vi "Lab Panel V5.25.vi"() -> ()   [LabVIEW 2017] (continued)
                n199 = local write "LAB03 TEMP"(w225) -> ()
                n200 = Unbundle(w202) -> ("id1"=→"LAB01-TP":bool, "id2"=→"LAB02-TP":bool, "id3"=→"LAB03-TP":bool, "id4"=→"LAB04-TP":bool, "id5"=→"LAB05-TP":bool)
                n201 = local read "TEMP LA05"() -> (w210:T9)
                n202 = local read "TEMP LA04"() -> (w217:T9)
                n203 = local read "TEMP LA02"() -> (w231:T9)
                n204 = local read "TEMP LA03"() -> (w224:T9)
                n205 = local read "TEMP LA01"() -> (w238:T9)
                n206 = Bundle(cluster=w224, "TL-1"=w222, "TN-1"=w221, "TL-2"=w220, "TN-2"=w219) -> (w223:T9)  [unwired: 4 in]
                n207 = Bundle(cluster=w238, "TL-1"=w237, "TN-1"=w236, "TL-2"=w235, "TN-2"=w234) -> (w233:T9)  [unwired: 4 in]
                n208 = Bundle(cluster=w231, "TL-1"=w229, "TN-1"=w228, "TL-2"=w227, "TN-2"=w226) -> (w230:T9)  [unwired: 4 in]
                n209 = Bundle(cluster=w217, "TL-1"=w216, "TN-1"=w215, "TL-2"=w214, "TN-2"=w213) -> (w212:T9)  [unwired: 4 in]
                n210 = Bundle(cluster=w210, "TL-1"=w209, "TN-1"=w208, "TL-2"=w207, "TN-2"=w206) -> (w205:T9)  [unwired: 4 in]
                n211 = local write "TEMP LA03"(w223) -> ()
                n212 = local write "TEMP LA01"(w233) -> ()
                n213 = local write "TEMP LA02"(w230) -> ()
                n214 = local write "TEMP LA05"(w205) -> ()
                n215 = local write "TEMP LA04"(w212) -> ()
              }
            }
            frame #2 {
              w252 = 0
              n216 = local read "LAB01 TEMP"() -> (w254:T12)
              n217 = local read "SIG LAB01-2"() -> (w249:T2)
              n218 = Unbundle By Name(w254) -> ("T1 Live"=w247:dbl, "T1 Neut"=w246:dbl, "T2 Live"=w245:dbl, "T2 Neut"=w244:dbl)  [unwired: 2 out]
              n219 = local read "SIG LAB01-1"() -> (w251:T2)
              n220 = local read "TEMP LA01"() -> (w255:T9)
              n221 = Bundle By Name(cluster=w255, "TL-1"=w247, "TN-1"=w246, "TL-2"=w245, "TN-2"=w244, "TL -1COUNT"=w252, "TN-1 COUNT"=w252, "TL-2 COUNT"=w252, "TN-2 COUNT"=w252) -> (w253:T9)
              n222 = Bundle(cluster=w251, "Tmp Live"=w247, "Tmp Neut"=w246) -> (w250:T2)  [unwired: 3 in]
              n223 = Bundle(cluster=w249, "Tmp Live"=w245, "Tmp Neut"=w244) -> (w248:T2)  [unwired: 3 in]
              n224 = local write "SIG LAB01-2"(w248) -> ()
              n225 = local write "SIG LAB01-1"(w250) -> ()
              n226 = local write "TEMP LA01"(w253) -> ()
            }
            frame #3 {
              w264 = 0
              n227 = local read "LAB02 TEMP"() -> (w266:T12)
              n228 = Unbundle By Name(w266) -> ("T1 Live"=w259:dbl, "T1 Neut"=w258:dbl, "T2 Live"=w257:dbl, "T2 Neut"=w256:dbl)  [unwired: 2 out]
              n229 = local read "SIG LAB02-1"() -> (w263:T2)
              n230 = local read "SIG LAB02-2"() -> (w262:T2)
              n231 = local read "TEMP LA02"() -> (w267:T9)
              n232 = Bundle By Name(cluster=w267, "TL-1"=w259, "TN-1"=w258, "TL-2"=w257, "TN-2"=w256, "TL -1COUNT"=w264, "TN-1 COUNT"=w264, "TL-2 COUNT"=w264, "TN-2 COUNT"=w264) -> (w265:T9)
              n233 = Bundle(cluster=w262, "Tmp Live"=w257, "Tmp Neut"=w256) -> (w260:T2)  [unwired: 3 in]
              n234 = Bundle(cluster=w263, "Tmp Live"=w259, "Tmp Neut"=w258) -> (w261:T2)  [unwired: 3 in]
              n235 = local write "TEMP LA02"(w265) -> ()
              n236 = local write "SIG LAB02-1"(w261) -> ()
              n237 = local write "SIG LAB02-2"(w260) -> ()
            }
            frame #4 {
              w276 = 0
              n238 = local read "LAB03 TEMP"() -> (w278:T12)
              n239 = Unbundle By Name(w278) -> ("T1 Live"=w271:dbl, "T1 Neut"=w270:dbl, "T2 Live"=w269:dbl, "T2 Neut"=w268:dbl)  [unwired: 2 out]
              n240 = local read "SIG LAB03-1"() -> (w275:T2)
              n241 = local read "SIG LAB03-2"() -> (w274:T2)
              n242 = local read "TEMP LA03"() -> (w279:T9)
              n243 = Bundle By Name(cluster=w279, "TL-1"=w271, "TN-1"=w270, "TL-2"=w269, "TN-2"=w268, "TL -1COUNT"=w276, "TN-1 COUNT"=w276, "TL-2 COUNT"=w276, "TN-2 COUNT"=w276) -> (w277:T9)
              n244 = Bundle(cluster=w274, "Tmp Live"=w269, "Tmp Neut"=w268) -> (w272:T2)  [unwired: 3 in]
              n245 = Bundle(cluster=w275, "Tmp Live"=w271, "Tmp Neut"=w270) -> (w273:T2)  [unwired: 3 in]
              n246 = local write "TEMP LA03"(w277) -> ()
              n247 = local write "SIG LAB03-2"(w272) -> ()
              n248 = local write "SIG LAB03-1"(w273) -> ()
            }
            frame #5 {
              w288 = 0
              n249 = local read "LAB04 TEMP"() -> (w290:T12)
              n250 = Unbundle By Name(w290) -> ("T1 Live"=w283:dbl, "T1 Neut"=w282:dbl, "T2 Live"=w281:dbl, "T2 Neut"=w280:dbl)  [unwired: 2 out]
              n251 = local read "SIG LAB04-2"() -> (w286:T2)
              n252 = local read "SIG LAB04-1"() -> (w287:T2)
              n253 = local read "TEMP LA04"() -> (w291:T9)
              n254 = Bundle By Name(cluster=w291, "TL-1"=w283, "TN-1"=w282, "TL-2"=w281, "TN-2"=w280, "TL -1COUNT"=w288, "TN-1 COUNT"=w288, "TL-2 COUNT"=w288, "TN-2 COUNT"=w288) -> (w289:T9)
              n255 = Bundle(cluster=w286, "Tmp Live"=w281, "Tmp Neut"=w280) -> (w284:T2)  [unwired: 3 in]
              n256 = Bundle(cluster=w287, "Tmp Live"=w283, "Tmp Neut"=w282) -> (w285:T2)  [unwired: 3 in]
              n257 = local write "SIG LAB04-2"(w284) -> ()
              n258 = local write "TEMP LA04"(w289) -> ()
              n259 = local write "SIG LAB04-1"(w285) -> ()
            }
            frame #6 {
              w300 = 0
              n260 = local read "LAB05 TEMP"() -> (w302:T12)
              n261 = Unbundle By Name(w302) -> ("T1 Live"=w295:dbl, "T1 Neut"=w294:dbl, "T2 Live"=w293:dbl, "T2 Neut"=w292:dbl)  [unwired: 2 out]
              n262 = local read "SIG LAB05-2"() -> (w298:T2)
              n263 = local read "SIG LAB05-1"() -> (w299:T2)
              n264 = local read "TEMP LA05"() -> (w303:T9)
              n265 = Bundle By Name(cluster=w303, "TL-1"=w295, "TN-1"=w294, "TL-2"=w293, "TN-2"=w292, "TL -1COUNT"=w300, "TN-1 COUNT"=w300, "TL-2 COUNT"=w300, "TN-2 COUNT"=w300) -> (w301:T9)
              n266 = Bundle(cluster=w298, "Tmp Live"=w293, "Tmp Neut"=w292) -> (w296:T2)  [unwired: 3 in]
              n267 = Bundle(cluster=w299, "Tmp Live"=w295, "Tmp Neut"=w294) -> (w297:T2)  [unwired: 3 in]
              n268 = local write "SIG LAB05-2"(w296) -> ()
              n269 = local write "SIG LAB05-1"(w297) -> ()
              n270 = local write "TEMP LA05"(w301) -> ()
            }
          }
        }
        frame #10 {
          # "create analog task"
          n271 = local read "AI Task0"() -> (w310:dbl)
          n272 = local read "AI Task1"() -> (w309:dbl)
          n273 = local read "AI Task2"() -> (w308:dbl)
          n274 = call "sub vi - AI USB4704 (3)  Create Task v2.vi"("Task In 0"=w310, "Task In 1"=w309, "Task In 2"=w308) -> ("TASK USB 0"=→"AI Task0":i32, "TASK USB 1"=→"AI Task1":i32, "TASK USB 2"=→"AI Task2":i32, "AI Task Er"=→"AI Task":bool)  [unwired: 8 in, 1 out]
        }
        frame #11 {
          # "enable front panel, all settings done"
          n275 = property on="Tab Control 2" class="TabCtl (strict)"("DisabledEnum"=T16."Enabled" ("Disabled")) -> ()  [unwired: 2 in, 2 out]
          n276 = property on="Tab Control 2" class="TabCtl (strict)"("Value"=0) -> ()  [unwired: 2 in, 2 out]
        }
        frame #12 {
          n277 = property on="Tab Control 2" class="TabCtl (strict)"("Value"=0) -> ()  [unwired: 2 in, 2 out]
        }
      }
    }
    frame #2 {
      n278 = node-c288("loop  delay(mS)") -> (w316:T18)  [unwired: 3 in]
      n279 = timed-loop {
        timing: w316 -> [_]
        timing-out: [_] -> w315
        i -> [w342]
        stop <- w317 stop-if-true
        n280 = node-c288() -> ()  [unwired: 1 in, 1 out]
        n281 = local read "Resets Done"() -> (w321:dbl)
        n282 = Greater?(x=w321, y=50) -> (0:w318:bool)
        n283 = local read "SELECT LAB05-2"() -> (w322:T3)
        n284 = local read "SELECT LAB05-1"() -> (w323:T3)
        n285 = local read "SELECT LAB04-2"() -> (w324:T3)
        n286 = Or(x=w318, y="stop") -> (x .or. y?=w317:bool)
        n287 = local read "SELECT LAB03-1"() -> (w327:T3)
        n288 = local read "SELECT LAB02-2"() -> (w328:T3)
        n289 = local read "SELECT LAB01-1"() -> (w331:T3)
        n290 = local read "SELECT LAB03-2"() -> (w326:T3)
        n291 = local read "SELECT LAB01-2"() -> (w330:T3)
        n292 = local read "SELECT LAB04-1"() -> (w325:T3)
        n293 = local read "SELECT LAB02-1"() -> (w329:T3)
        n294 = local read "run lab03-2"() -> (w336:bool)
        n295 = local read "run lab04-1"() -> (w335:bool)
        n296 = local read "run lab05-1"() -> (w333:bool)
        n297 = local read "run lab04-2"() -> (w334:bool)
        n298 = local read "run lab05-2"() -> (w332:bool)
        n299 = local read "run lab03-1"() -> (w337:bool)
        n300 = local read "run lab02-2"() -> (w338:bool)
        n301 = local read "run lab02-1"() -> (w339:bool)
        n302 = local read "run lab01-1"() -> (w341:bool)
        n303 = local read "run lab01-2"() -> (w340:bool)
        n304 = global write "Global display 1.vi" "stop disp"(w317) -> ()
        n305 = stacked-sequence {
          seq-local: [_ w408 _ _ _ _ _ _ _ _ _ _ _ _ _ _ _ _ _ _ _ _ _ _] -> [_ _ _ _ _ w2509 _ _ _ _ _ _ _ _ _ _ _ _ _ _ _ _ _ _]
          seq-local: [_ w407 _ _ _ _ _ _ _ _ _ _ _ _ _ _ _ _ _ _ _ _ _ _] -> [_ _ _ _ _ w2508 _ _ _ _ _ _ _ _ _ _ _ _ _ _ _ _ _ _]
          seq-local: [_ w394 _ _ _ _ _ _ _ _ _ _ _ _ _ _ _ _ _ _ _ _ _ _] -> [_ _ _ _ _ w2507 _ _ _ _ _ _ _ _ _ _ _ _ _ _ _ _ _ _]
          seq-local: [_ w393 _ _ _ _ _ _ _ _ _ _ _ _ _ _ _ _ _ _ _ _ _ _] -> [_ _ _ _ _ w2506 _ _ _ _ _ _ _ _ _ _ _ _ _ _ _ _ _ _]
          seq-local: [_ w392 _ _ _ _ _ _ _ _ _ _ _ _ _ _ _ _ _ _ _ _ _ _] -> [_ _ _ _ _ w2505 _ _ _ _ _ _ _ _ _ _ _ _ _ _ _ _ _ _]
          seq-local: [_ w391 _ _ _ _ _ _ _ _ _ _ _ _ _ _ _ _ _ _ _ _ _ _] -> [_ _ _ _ _ w2504 _ _ _ _ _ _ _ _ _ _ _ _ _ _ _ _ _ _]
          seq-local: [_ w390 _ _ _ _ _ _ _ _ _ _ _ _ _ _ _ _ _ _ _ _ _ _] -> [_ _ _ _ _ w2503 _ _ _ _ _ _ _ _ _ _ _ _ _ _ _ _ _ _]
          seq-local: [_ w389 _ _ _ _ _ _ _ _ _ _ _ _ _ _ _ _ _ _ _ _ _ _] -> [_ _ _ _ _ w2502 _ _ _ _ _ _ _ _ _ _ _ _ _ _ _ _ _ _]
          seq-local: [_ w388 _ _ _ _ _ _ _ _ _ _ _ _ _ _ _ _ _ _ _ _ _ _] -> [_ _ _ _ _ w2501 _ _ _ _ _ _ _ _ _ _ _ _ _ _ _ _ _ _]
          seq-local: [_ w387 _ _ _ _ _ _ _ _ _ _ _ _ _ _ _ _ _ _ _ _ _ _] -> [_ _ _ _ _ w2500 _ _ _ _ _ _ _ _ _ _ _ _ _ _ _ _ _ _]
          seq-local: [_ _ _ _ _ _ _ _ _ _ _ w3640 _ _ _ _ _ _ _ _ _ _ _ _] -> [_ _ _ _ _ _ _ _ _ _ _ _ w3661 _ _ _ _ _ _ _ _ _ _ _]
          tunnel: w341 -> [_ _ w424 w672 w2099 w2529 w2844 w3331 _ _ _ _ _ w3946 _ w4903 _ _ w5190 w5493 w5674 _ _ _]
          tunnel: w340 -> [_ _ w423 w670 w2098 w2528 w2845 w3330 _ _ _ _ _ w3945 _ w4901 _ _ w5189 w5492 w5672 _ _ _]
          tunnel: w339 -> [_ _ w422 w668 w2097 w2527 w2843 w3329 _ _ _ _ _ w3944 _ w4899 _ _ w5188 w5491 w5671 _ _ _]
          tunnel: w338 -> [_ _ w421 w666 w2096 w2526 w2842 w3328 _ _ _ _ _ w3943 _ w4897 _ _ w5187 w5490 w5670 _ _ _]
          tunnel: w337 -> [_ _ w420 w664 w2095 w2525 w2841 w3327 _ _ _ _ _ w3942 _ w4895 _ _ w5186 w5489 w5669 _ _ _]
          tunnel: w336 -> [_ _ w419 w662 w2094 w2524 w2840 w3326 _ _ _ _ _ w3941 _ w4893 _ _ w5185 w5488 w5668 _ _ _]
          tunnel: w335 -> [_ _ w418 w660 w2093 w2523 w2839 w3325 _ _ _ _ _ w3940 _ w4891 _ _ w5184 w5487 w5667 _ _ _]
          tunnel: w334 -> [_ _ w417 w658 w2092 w2522 w2838 w3324 _ _ _ _ _ w3939 _ w4889 _ _ w5183 w5486 w5666 _ _ _]
          tunnel: w333 -> [_ _ w416 w656 w2091 w2521 w2837 w3323 _ _ _ _ _ w3938 _ w4887 _ _ w5182 w5485 w5665 _ _ _]
          tunnel: w332 -> [_ _ w415 w654 w2090 w2520 w2836 w3322 _ _ _ _ _ w3937 _ w4885 _ _ w5181 w5484 w5664 _ _ _]
          tunnel: w331 -> [_ _ _ w671 w2089 w2519 _ _ _ _ _ _ _ _ _ w4905 _ _ _ _ _ w6018 _ _]
          tunnel: w330 -> [_ _ _ w669 w2088 w2518 _ _ _ _ _ _ _ _ _ w4900 _ _ _ _ _ w6017 _ _]
          tunnel: w329 -> [_ _ _ w667 w2087 w2517 _ _ _ _ _ _ _ _ _ w4898 _ _ _ _ _ w6016 _ _]
          tunnel: w328 -> [_ _ _ w665 w2086 w2516 _ _ _ _ _ _ _ _ _ w4896 _ _ _ _ _ w6015 _ _]
          tunnel: w327 -> [_ _ _ w663 w2085 w2515 _ _ _ _ _ _ _ _ _ w4894 _ _ _ _ _ w6014 _ _]
          tunnel: w326 -> [_ _ _ w661 w2084 w2514 _ _ _ _ _ _ _ _ _ w4892 _ _ _ _ _ w6013 _ _]
          tunnel: w325 -> [_ _ _ w659 w2083 w2513 _ _ _ _ _ _ _ _ _ w4890 _ _ _ _ _ w6012 _ _]
          tunnel: w324 -> [_ _ _ w657 w2082 w2512 _ _ _ _ _ _ _ _ _ w4888 _ _ _ _ _ w6011 _ _]
          tunnel: w323 -> [_ _ _ w655 w2081 w2511 _ _ _ _ _ _ _ _ _ w4886 _ _ _ _ _ w6010 _ _]
          tunnel: w322 -> [_ _ _ w653 w2080 w2510 _ _ _ _ _ _ _ _ _ w4884 _ _ _ _ _ w6009 _ _]
          tunnel: w318 -> [_ _ _ _ _ _ _ _ _ _ _ _ _ _ _ _ _ _ _ _ _ _ _ w6071]
          tunnel: w317 -> [_ _ _ _ _ _ _ _ _ _ _ _ _ _ _ _ _ _ _ _ _ _ _ w6070]
          frame #0 {
            w350 = FALSE
            w355 = 0.5
            # "set up cycle control"
            n306 = local read "jig cycle"() -> (w354:dbl)
            n307 = local read "Amps Fail level"() -> (w348:dbl)
            n308 = local read "Simulate"() -> (w345:bool)
            n309 = Divide(x="JIG ON TIME (S)", y=w355) -> (x/y=→"on loops":dbl)
            n310 = Divide(x="JIG OFF TIME (S)", y=w355) -> (x/y=→"off loops":dbl)
            n311 = Increment(x=w354) -> (x+1=w353:dbl)
            n312 = local write "Simulate IND"(w345) -> ()
            n313 = global write "Global display 3.vi" "Amps Fail"(w348) -> ()
            n314 = local write "TEMP"(w350) -> ()
            n315 = local write "AI"(w350) -> ()
            n316 = local read "Network Directory"() -> (w347:path)
            n317 = local write "jig cycle"(w353) -> ()
            n318 = call "sub vi - check network dir v2.vi"("PATH"=w347) -> ("error"=w346:bool)  [unwired: 10 in]
            n319 = local write "network error"(w346) -> ()
            n320 = global write "Global display 3.vi" "network drive"(w346) -> ()
            n321 = event shown="[1] \"ADMIN\": Value Change" {
              selector: _ -> [_ _]
              dyn-events: _ -> [_ _]
              timeout: 10 -> [_ _]
              event Timeout {
                n322 = event-data() -> ()  [unwired: 1 in, 3 out]
              }
              event "ADMIN": Value Change {
                n323 = event-data() -> ()  [unwired: 1 in, 6 out]
                n324 = stacked-sequence {
                  seq-local: [_ w359 _] -> [_ _ w360]
                  frame #0 {
                    n325 = global write "Global 1.vi" "password"("9949") -> ()
                  }
                  frame #1 {
                    n326 = call "sub vi - password 1.vi"() -> ("RESULT"=w359:bool)  [unwired: 11 in]
                  }
                  frame #2 {
                    w362 = FALSE
                    n327 = property on="Tab Control 2" class="TabCtl (strict)"() -> ("Pages"=w366:refnum<vi>[])  [unwired: 2 in, 2 out]
                    n328 = Select(t=TRUE, s=w360, f=w362) -> (s? t:f=w361:bool)
                    n329 = Index Array(array=w366, index=8) -> (element=w364:refnum<vi>)
                    n330 = property class="Page"(reference=w364, "PageVis"=w361) -> ()  [unwired: 1 in, 2 out]
                    n331 = local write "ADMIN"(w362) -> ()
                  }
                }
              }
            }
          }
          frame #1 {
            w404 = 60.0
            # "convert temperature rise minutes to cycles"
            n332 = local read "SET LAB05-2"() -> (w368:T5)
            n333 = local read "SET LAB05-1"() -> (w370:T5)
            n334 = local read "SET LAB04-2"() -> (w372:T5)
            n335 = local read "SET LAB01-1"() -> (w386:T5)
            n336 = local read "SET LAB01-2"() -> (w384:T5)
            n337 = local read "SET LAB02-2"() -> (w380:T5)
            n338 = local read "SET LAB04-1"() -> (w374:T5)
            n339 = local read "SET LAB03-1"() -> (w378:T5)
            n340 = local read "SET LAB03-2"() -> (w376:T5)
            n341 = local read "SET LAB02-1"() -> (w382:T5)
            n342 = local read "JIG OFF TIME (S)"() -> (w409:dbl)
            n343 = local read "JIG ON TIME (S)"() -> (w410:dbl)
            n344 = Unbundle(w368) -> ("T-RISE mins"=w367:dbl)  [unwired: 4 out]
            n345 = Unbundle(w370) -> ("T-RISE mins"=w369:dbl)  [unwired: 4 out]
            n346 = Unbundle(w386) -> ("T-RISE mins"=w385:dbl)  [unwired: 4 out]
            n347 = Unbundle(w372) -> ("T-RISE mins"=w371:dbl)  [unwired: 4 out]
            n348 = Unbundle(w384) -> ("T-RISE mins"=w383:dbl)  [unwired: 4 out]
            n349 = Unbundle(w382) -> ("T-RISE mins"=w381:dbl)  [unwired: 4 out]
            n350 = Unbundle(w374) -> ("T-RISE mins"=w373:dbl)  [unwired: 4 out]
            n351 = Unbundle(w380) -> ("T-RISE mins"=w379:dbl)  [unwired: 4 out]
            n352 = Unbundle(w376) -> ("T-RISE mins"=w375:dbl)  [unwired: 4 out]
            n353 = Unbundle(w378) -> ("T-RISE mins"=w377:dbl)  [unwired: 4 out]
            n354 = Add(x=w410, y=w409) -> (x+y=w403:dbl)
            n355 = Multiply(x=w404, y=w375) -> (x*y=w399:dbl)
            n356 = Multiply(x=w404, y=w373) -> (x*y=w398:dbl)
            n357 = Multiply(x=w404, y=w371) -> (x*y=w397:dbl)
            n358 = Multiply(x=w404, y=w369) -> (x*y=w396:dbl)
            n359 = Multiply(x=w404, y=w367) -> (x*y=w395:dbl)
            n360 = Multiply(x=w404, y=w383) -> (x*y=w405:dbl)
            n361 = Multiply(x=w404, y=w377) -> (x*y=w400:dbl)
            n362 = Multiply(x=w404, y=w385) -> (x*y=w406:dbl)
            n363 = Multiply(x=w404, y=w381) -> (x*y=w402:dbl)
            n364 = Multiply(x=w404, y=w379) -> (x*y=w401:dbl)
            n365 = Divide(x=w396, y=w403) -> (x/y=w388:dbl)
            n366 = Divide(x=w397, y=w403) -> (x/y=w389:dbl)
            n367 = Divide(x=w398, y=w403) -> (x/y=w390:dbl)
            n368 = Divide(x=w395, y=w403) -> (x/y=w387:dbl)
            n369 = Divide(x=w400, y=w403) -> (x/y=w392:dbl)
            n370 = Divide(x=w406, y=w403) -> (x/y=w408:dbl)
            n371 = Divide(x=w405, y=w403) -> (x/y=w407:dbl)
            n372 = Divide(x=w402, y=w403) -> (x/y=w394:dbl)
            n373 = Divide(x=w401, y=w403) -> (x/y=w393:dbl)
            n374 = Divide(x=w399, y=w403) -> (x/y=w391:dbl)
          }
          frame #2 {
            # "control cycle loops"
            n375 = local read "JIG OFF TIME (S)"() -> (w413:dbl)
            n376 = local read "JIG ON TIME (S)"() -> (w412:dbl)
            n377 = local read "jig cycle"() -> (w426:dbl)
            n378 = local read "on loops"() -> (w428:dbl)
            n379 = local read "off loops"() -> (w427:dbl)
            n380 = Add(x=w413, y=w412) -> (x+y=w411:dbl)
            n381 = Add(x=w428, y=w427) -> (x+y=w414:dbl)
            n382 = Greater Or Equal?(x=w426, y=w414) -> (x >= y?=w425:bool)
            n383 = case shown="True" w425 {
              tunnel: w424 -> [_ w462]
              tunnel: w423 -> [_ w461]
              tunnel: w422 -> [_ w460]
              tunnel: w421 -> [_ w459]
              tunnel: w420 -> [_ w458]
              tunnel: w419 -> [_ w457]
              tunnel: w418 -> [_ w456]
              tunnel: w417 -> [_ w455]
              tunnel: w416 -> [_ w454]
              tunnel: w415 -> [_ w453]
              tunnel: w411 -> [_ w452]
              frame False {
              }
              frame True {
                # "increment cycle value and convert cycles to minutes for temp rise"
                n384 = stacked-sequence {
                  frame #0 {
                    n385 = local read "Temp read loop"() -> (w465:dbl)
                    n386 = Increment(x=w465) -> (x+1=w464:dbl)
                    n387 = local write "Temp read loop"(w464) -> ()
                  }
                  frame #1 {
                    n388 = local read "Temp read loop"() -> (w466:dbl)
                    n389 = Greater?(x=w466, y=20) -> (0:w468:bool)
                    n390 = case shown="True" w468 {
                      frame False {
                      }
                      frame True {
                        n391 = local write "Temp read loop"(1) -> ()
                      }
                    }
                  }
                }
                n392 = local read "JIG RELAY CYCLES"() -> (w451:T8)
                n393 = local read "Temp read loop"() -> (→"Tp Up":dbl)
                n394 = Unbundle By Name(w451) -> ("LAB01-1"=w449:dbl, "LAB01-2"=w447:dbl, "LAB02-1"=w445:dbl, "LAB02-2"=w443:dbl, "LAB03-1"=w441:dbl, "LAB03-2"=w439:dbl, "LAB04-1"=w437:dbl, "LAB04-2"=w435:dbl, "LAB05-1"=w433:dbl, "LAB05-2"=w431:dbl)
                n395 = stacked-sequence {
                  tunnel: w462 -> [w480 _ _ _ _ _ _ _ _ _]
                  tunnel: w461 -> [_ w497 _ _ _ _ _ _ _ _]
                  tunnel: w460 -> [_ _ w514 _ _ _ _ _ _ _]
                  tunnel: w459 -> [_ _ _ w531 _ _ _ _ _ _]
                  tunnel: w458 -> [_ _ _ _ w548 _ _ _ _ _]
                  tunnel: w457 -> [_ _ _ _ _ w565 _ _ _ _]
                  tunnel: w456 -> [_ _ _ _ _ _ w582 _ _ _]
                  tunnel: w455 -> [_ _ _ _ _ _ _ w599 _ _]
                  tunnel: w454 -> [_ _ _ _ _ _ _ _ w616 _]
                  tunnel: w453 -> [_ _ _ _ _ _ _ _ _ w633]
                  tunnel: w452 -> [w477 w494 w511 w528 w545 w562 w579 w596 w613 w630]
                  tunnel: w449 -> [w471 _ _ _ _ _ _ _ _ _]
                  tunnel: [w470 _ _ _ _ _ _ _ _ _] -> w448
                  tunnel: w447 -> [_ w488 _ _ _ _ _ _ _ _]
                  tunnel: [_ w487 _ _ _ _ _ _ _ _] -> w446
                  tunnel: w445 -> [_ _ w505 _ _ _ _ _ _ _]
                  tunnel: [_ _ w504 _ _ _ _ _ _ _] -> w444
                  tunnel: w443 -> [_ _ _ w522 _ _ _ _ _ _]
                  tunnel: [_ _ _ w521 _ _ _ _ _ _] -> w442
                  tunnel: w441 -> [_ _ _ _ w539 _ _ _ _ _]
                  tunnel: [_ _ _ _ w538 _ _ _ _ _] -> w440
                  tunnel: w439 -> [_ _ _ _ _ w556 _ _ _ _]
                  tunnel: [_ _ _ _ _ w555 _ _ _ _] -> w438
                  tunnel: w437 -> [_ _ _ _ _ _ w573 _ _ _]
                  tunnel: [_ _ _ _ _ _ w572 _ _ _] -> w436
                  tunnel: w435 -> [_ _ _ _ _ _ _ w590 _ _]
                  tunnel: [_ _ _ _ _ _ _ w589 _ _] -> w434
                  tunnel: w433 -> [_ _ _ _ _ _ _ _ w607 _]
                  tunnel: [_ _ _ _ _ _ _ _ w606 _] -> w432
                  tunnel: w431 -> [_ _ _ _ _ _ _ _ _ w624]
                  tunnel: [_ _ _ _ _ _ _ _ _ w623] -> w430
                  frame #0 {
                    n396 = local read "DISP LAB01-1"() -> (w475:T4)
                    n397 = Unbundle(w475) -> ("CYCLE"=w476:dbl)  [unwired: 2 out]
                    n398 = case shown="True" w480 {
                      tunnel: w476 -> [w482 w486]
                      tunnel: [w482 w485] -> w474
                      tunnel: w471 -> [w481 w484]
                      tunnel: [w481 w483] -> w470
                      frame False {
                      }
                      frame True {
                        n399 = Increment(x=w484) -> (x+1=w483:dbl)
                        n400 = Increment(x=w486) -> (x+1=w485:dbl)
                      }
                    }
                    n401 = Multiply(x=w474, y=w477) -> (x*y=w478:dbl)
                    n402 = Divide(x=w478, y=60.0) -> (x/y=w473:dbl)
                    n403 = Bundle(cluster=w475, "CYCLE"=w474, "MINS"=w473) -> (w472:T4)  [unwired: 1 in]
                    n404 = local write "DISP LAB01-1"(w472) -> ()
                  }
                  frame #1 {
                    n405 = local read "DISP LAB01-2"() -> (w492:T4)
                    n406 = Unbundle(w492) -> ("CYCLE"=w493:dbl)  [unwired: 2 out]
                    n407 = case shown="True" w497 {
                      tunnel: w493 -> [w499 w503]
                      tunnel: [w499 w502] -> w490
                      tunnel: w488 -> [w498 w501]
                      tunnel: [w498 w500] -> w487
                      frame False {
                      }
                      frame True {
                        n408 = Increment(x=w501) -> (x+1=w500:dbl)
                        n409 = Increment(x=w503) -> (x+1=w502:dbl)
                      }
                    }
                    n410 = Multiply(x=w490, y=w494) -> (x*y=w495:dbl)
                    n411 = Divide(x=w495, y=60.0) -> (x/y=w489:dbl)
                    n412 = Bundle(cluster=w492, "CYCLE"=w490, "MINS"=w489) -> (w491:T4)  [unwired: 1 in]
                    n413 = local write "DISP LAB01-2"(w491) -> ()
                  }
                  frame #2 {
                    n414 = local read "DISP LAB02-1"() -> (w509:T4)
                    n415 = Unbundle(w509) -> ("CYCLE"=w510:dbl)  [unwired: 2 out]
                    n416 = case shown="True" w514 {
                      tunnel: [w516 w520] -> w507
                      tunnel: w510 -> [w516 w519]
                      tunnel: w505 -> [w515 w518]
                      tunnel: [w515 w517] -> w504
                      frame False {
                      }
                      frame True {
                        n417 = Increment(x=w518) -> (x+1=w517:dbl)
                        n418 = Increment(x=w519) -> (x+1=w520:dbl)
                      }
                    }
                    n419 = Multiply(x=w507, y=w511) -> (x*y=w512:dbl)
                    n420 = Divide(x=w512, y=60.0) -> (x/y=w506:dbl)
                    n421 = Bundle(cluster=w509, "CYCLE"=w507, "MINS"=w506) -> (w508:T4)  [unwired: 1 in]
                    n422 = local write "DISP LAB02-1"(w508) -> ()
                  }
                  frame #3 {
                    n423 = local read "DISP LAB02-2"() -> (w526:T4)
                    n424 = Unbundle(w526) -> ("CYCLE"=w527:dbl)  [unwired: 2 out]
                    n425 = case shown="True" w531 {
                      tunnel: [w533 w537] -> w525
                      tunnel: w527 -> [w533 w536]
                      tunnel: w522 -> [w532 w535]
                      tunnel: [w532 w534] -> w521
                      frame False {
                      }
                      frame True {
                        n426 = Increment(x=w535) -> (x+1=w534:dbl)
                        n427 = Increment(x=w536) -> (x+1=w537:dbl)
                      }
                    }
                    n428 = Multiply(x=w525, y=w528) -> (x*y=w529:dbl)
                    n429 = Divide(x=w529, y=60.0) -> (x/y=w524:dbl)
                    n430 = Bundle(cluster=w526, "CYCLE"=w525, "MINS"=w524) -> (w523:T4)  [unwired: 1 in]
                    n431 = local write "DISP LAB02-2"(w523) -> ()
                  }
                  frame #4 {
                    n432 = local read "DISP LAB03-1"() -> (w543:T4)
                    n433 = Unbundle(w543) -> ("CYCLE"=w544:dbl)  [unwired: 2 out]
                    n434 = case shown="True" w548 {
                      tunnel: [w550 w554] -> w540
                      tunnel: w544 -> [w550 w553]
                      tunnel: w539 -> [w549 w552]
                      tunnel: [w549 w551] -> w538
                      frame False {
                      }
                      frame True {
                        n435 = Increment(x=w552) -> (x+1=w551:dbl)
                        n436 = Increment(x=w553) -> (x+1=w554:dbl)
                      }
                    }
                    n437 = Multiply(x=w540, y=w545) -> (x*y=w546:dbl)
                    n438 = Divide(x=w546, y=60.0) -> (x/y=w541:dbl)
                    n439 = Bundle(cluster=w543, "CYCLE"=w540, "MINS"=w541) -> (w542:T4)  [unwired: 1 in]
                    n440 = local write "DISP LAB03-1"(w542) -> ()
                  }
                  frame #5 {
                    n441 = local read "DISP LAB03-2"() -> (w560:T4)
                    n442 = Unbundle(w560) -> ("CYCLE"=w561:dbl)  [unwired: 2 out]
                    n443 = case shown="True" w565 {
                      tunnel: [w567 w571] -> w559
                      tunnel: w561 -> [w567 w570]
                      tunnel: w556 -> [w566 w569]
                      tunnel: [w566 w568] -> w555
                      frame False {
                      }
                      frame True {
                        n444 = Increment(x=w569) -> (x+1=w568:dbl)
                        n445 = Increment(x=w570) -> (x+1=w571:dbl)
                      }
                    }
                    n446 = Multiply(x=w559, y=w562) -> (x*y=w563:dbl)
                    n447 = Divide(x=w563, y=60.0) -> (x/y=w558:dbl)
                    n448 = Bundle(cluster=w560, "CYCLE"=w559, "MINS"=w558) -> (w557:T4)  [unwired: 1 in]
                    n449 = local write "DISP LAB03-2"(w557) -> ()
                  }
                  frame #6 {
                    n450 = local read "DISP LAB04-1"() -> (w577:T4)
                    n451 = Unbundle(w577) -> ("CYCLE"=w578:dbl)  [unwired: 2 out]
                    n452 = case shown="True" w582 {
                      tunnel: [w584 w588] -> w575
                      tunnel: w578 -> [w584 w587]
                      tunnel: w573 -> [w583 w586]
                      tunnel: [w583 w585] -> w572
                      frame False {
                      }
                      frame True {
                        n453 = Increment(x=w586) -> (x+1=w585:dbl)
                        n454 = Increment(x=w587) -> (x+1=w588:dbl)
                      }
                    }
                    n455 = Multiply(x=w575, y=w579) -> (x*y=w580:dbl)
                    n456 = Divide(x=w580, y=60.0) -> (x/y=w574:dbl)
                    n457 = Bundle(cluster=w577, "CYCLE"=w575, "MINS"=w574) -> (w576:T4)  [unwired: 1 in]
                    n458 = local write "DISP LAB04-1"(w576) -> ()
                  }
                  frame #7 {
                    n459 = local read "DISP LAB04-2"() -> (w594:T4)
                    n460 = Unbundle(w594) -> ("CYCLE"=w595:dbl)  [unwired: 2 out]
                    n461 = case shown="True" w599 {
                      tunnel: [w601 w605] -> w592
                      tunnel: w595 -> [w601 w604]
                      tunnel: w590 -> [w600 w603]
                      tunnel: [w600 w602] -> w589
                      frame False {
                      }
                      frame True {
                        n462 = Increment(x=w603) -> (x+1=w602:dbl)
                        n463 = Increment(x=w604) -> (x+1=w605:dbl)
                      }
                    }
                    n464 = Multiply(x=w592, y=w596) -> (x*y=w598:dbl)
                    n465 = Divide(x=w598, y=60.0) -> (x/y=w591:dbl)
                    n466 = Bundle(cluster=w594, "CYCLE"=w592, "MINS"=w591) -> (w593:T4)  [unwired: 1 in]
                    n467 = local write "DISP LAB04-2"(w593) -> ()
                  }
                  frame #8 {
                    n468 = local read "DISP LAB05-1"() -> (w611:T4)
                    n469 = Unbundle(w611) -> ("CYCLE"=w612:dbl)  [unwired: 2 out]
                    n470 = case shown="True" w616 {
                      tunnel: [w618 w622] -> w609
                      tunnel: w612 -> [w618 w621]
                      tunnel: w607 -> [w617 w620]
                      tunnel: [w617 w619] -> w606
                      frame False {
                      }
                      frame True {
                        n471 = Increment(x=w620) -> (x+1=w619:dbl)
                        n472 = Increment(x=w621) -> (x+1=w622:dbl)
                      }
                    }
                    n473 = Multiply(x=w609, y=w613) -> (x*y=w614:dbl)
                    n474 = Divide(x=w614, y=60.0) -> (x/y=w608:dbl)
                    n475 = Bundle(cluster=w611, "CYCLE"=w609, "MINS"=w608) -> (w610:T4)  [unwired: 1 in]
                    n476 = local write "DISP LAB05-1"(w610) -> ()
                  }
                  frame #9 {
                    n477 = local read "DISP LAB05-2"() -> (w629:T4)
                    n478 = Unbundle(w629) -> ("CYCLE"=w628:dbl)  [unwired: 2 out]
                    n479 = case shown="True" w633 {
                      tunnel: [w635 w639] -> w627
                      tunnel: w628 -> [w635 w638]
                      tunnel: w624 -> [w634 w637]
                      tunnel: [w634 w636] -> w623
                      frame False {
                      }
                      frame True {
                        n480 = Increment(x=w637) -> (x+1=w636:dbl)
                        n481 = Increment(x=w638) -> (x+1=w639:dbl)
                      }
                    }
                    n482 = Multiply(x=w627, y=w630) -> (x*y=w631:dbl)
                    n483 = Divide(x=w631, y=60.0) -> (x/y=w626:dbl)
                    n484 = Bundle(cluster=w629, "CYCLE"=w627, "MINS"=w626) -> (w625:T4)  [unwired: 1 in]
                    n485 = local write "DISP LAB05-2"(w625) -> ()
                  }
                }
                n486 = local write "jig cycle"(0) -> ()
                n487 = Bundle By Name(cluster=w451, "LAB01-1"=w448, "LAB01-2"=w446, "LAB02-1"=w444, "LAB02-2"=w442, "LAB03-1"=w440, "LAB03-2"=w438, "LAB04-1"=w436, "LAB04-2"=w434, "LAB05-1"=w432, "LAB05-2"=w430) -> (w450:T8)
                n488 = local write "JIG RELAY CYCLES"(w450) -> ()
              }
            }
          }
          frame #3 {
            # "START & STOP test RUN switch change, start test if true and stop test if false"
            n489 = Get Date/Time In Seconds() -> (seconds since 1Jan1904=w651:timestamp)
            n490 = local read "C drive data root dir"() -> (w644:path)
            n491 = Format Date/Time String(time format string (%c)="%b\\%a%d", seconds (now)=w651) -> (date/time string=w675:string)  [unwired: 1 in]
            n492 = Format Date/Time String(time format string (%c)="%H%M", seconds (now)=w651) -> (date/time string=w673:string)  [unwired: 1 in]
            n493 = Format Date/Time String(time format string (%c)="LabPanel%Y", seconds (now)=w651) -> (date/time string=w650:string)  [unwired: 1 in]
            n494 = Path To String(path=w644) -> (string=w647:string)
            n495 = global write "Global 1.vi" "C drive root path"(w644) -> ()
            n496 = local read "Ref deg C"() -> (w640:dbl)
            n497 = Concatenate Strings(w647, "\\") -> (w645:string)
            n498 = event shown="[1] \"RUN LAB01-1\": Value Change" {
              selector: _ -> [_ _ _ _ _ _ _ _ _ _ _]
              dyn-events: _ -> [_ _ _ _ _ _ _ _ _ _ _]
              timeout: 10 -> [_ _ _ _ _ _ _ _ _ _ _]
              tunnel: w645 -> [_ w688 w828 w969 w1109 w1249 w1389 w1529 w1669 w1809 w1950]
              tunnel: w675 -> [_ w687 w827 w968 w1108 w1248 w1388 w1528 w1668 w1808 w1949]
              tunnel: w673 -> [_ w685 w826 w967 w1107 w1247 w1387 w1527 w1667 w1807 w1948]
              tunnel: w671 -> [_ w686 _ _ _ _ _ _ _ _ _]
              tunnel: w672 -> [_ _ _ _ _ _ _ _ _ _ _]
              tunnel: w670 -> [_ _ _ _ _ _ _ _ _ _ _]
              tunnel: w669 -> [_ _ w825 _ _ _ _ _ _ _ _]
              tunnel: w668 -> [_ _ _ _ _ _ _ _ _ _ _]
              tunnel: w667 -> [_ _ _ w966 _ _ _ _ _ _ _]
              tunnel: w666 -> [_ _ _ _ _ _ _ _ _ _ _]
              tunnel: w665 -> [_ _ _ _ w1106 _ _ _ _ _ _]
              tunnel: w664 -> [_ _ _ _ _ _ _ _ _ _ _]
              tunnel: w663 -> [_ _ _ _ _ w1246 _ _ _ _ _]
              tunnel: w662 -> [_ _ _ _ _ _ _ _ _ _ _]
              tunnel: w661 -> [_ _ _ _ _ _ w1386 _ _ _ _]
              tunnel: w660 -> [_ _ _ _ _ _ _ _ _ _ _]
              tunnel: w659 -> [_ _ _ _ _ _ _ w1526 _ _ _]
              tunnel: w658 -> [_ _ _ _ _ _ _ _ _ _ _]
              tunnel: w657 -> [_ _ _ _ _ _ _ _ w1666 _ _]
              tunnel: w656 -> [_ _ _ _ _ _ _ _ _ _ _]
              tunnel: w655 -> [_ _ _ _ _ _ _ _ _ w1806 _]
              tunnel: w654 -> [_ _ _ _ _ _ _ _ _ _ _]
              tunnel: w653 -> [_ _ _ _ _ _ _ _ _ _ w1947]
              tunnel: w650 -> [_ w684 w824 w965 w1105 w1245 w1385 w1525 w1665 w1805 w1946]
              tunnel: [_ w683 w823 w964 w1104 w1244 w1384 w1524 w1664 w1804 w1945] -> w648
              tunnel: "RESET CYCLES TO ZERO?" -> [_ w682 w821 w962 w1102 w1242 w1382 w1522 w1662 w1802 w1943]
              tunnel: "YES" -> [_ w681 w820 w961 w1101 w1241 w1381 w1521 w1661 w1801 w1942]
              tunnel: "NO" -> [_ w680 w819 w960 w1100 w1240 w1380 w1520 w1660 w1800 w1941]
              tunnel: w640 -> [_ w677 w818 w958 w1099 w1239 w1379 w1519 w1659 w1799 w1939]
              event Timeout {
                n499 = event-data() -> ()  [unwired: 1 in, 3 out]
              }
              event "RUN LAB01-1": Value Change {
                n500 = event-data() -> ("NewVal"=w678:bool)  [unwired: 1 in, 5 out]
                n501 = local read "SIG LAB01-1"() -> (w679:T2)
                n502 = local write "run lab01-1"(w678) -> ()
                n503 = case shown="True" w678 {
                  tunnel: w688 -> [_ w726]
                  tunnel: w687 -> [_ w725]
                  tunnel: w686 -> [w690 w724]
                  tunnel: w685 -> [_ w723]
                  tunnel: w684 -> [_ w722]
                  tunnel: [w689 w721] -> w683
                  tunnel: w682 -> [_ w720]
                  tunnel: w681 -> [_ w719]
                  tunnel: w680 -> [_ w718]
                  tunnel: w679 -> [_ w717]
                  tunnel: w677 -> [_ w716]
                  frame False {
                    # "stop test"
                    n504 = stacked-sequence {
                      tunnel: w690 -> [_ w702 _]
                      tunnel: [_ w694 _] -> w689
                      frame #0 {
                        n505 = local read "DISP LAB01-1"() -> (w693:T4)
                        n506 = Bundle(cluster=w693, "STATUS"="STOP") -> (w691:T4)  [unwired: 2 in]
                        n507 = local write "DISP LAB01-1"(w691) -> ()
                      }
                      frame #1 {
                        n508 = local read "DISP LAB01-1"() -> (w701:T4)
                        n509 = Unbundle(w701) -> ("CYCLE"=w699:dbl, "MINS"=w700:dbl)  [unwired: 1 out]
                        n510 = case shown="\"CYCLE TEST\"" w702 {
                          tunnel: w700 -> [_ _ w709]
                          tunnel: w699 -> [w707 w708 _]
                          tunnel: [w707 w708 w709] -> w698
                          frame "CHART TEST", Default {
                          }
                          frame "CYCLE TEST" {
                          }
                          frame "T-RISE TEST" {
                          }
                        }
                        n511 = local read "TDMS LAB01-1"() -> (w706:refnum<k34>)
                        n512 = Build Array("STOPPED") -> (w703:string[])
                        n513 = Build Array(w698) -> (w697:dbl[])
                        n514 = TDMS Write(0:w706, 5:"TEST RESULT", 7:w703, 9:w697) -> (4:w695:refnum<k34>, 15:w696:errorcluster)  [unwired: 2 in, 2 out]
                        n515 = TDMS Close(8:w696, 11:w695) -> (0:w694:errorcluster)  [unwired: 1 out]
                      }
                      frame #2 {
                        n516 = stacked-sequence {
                          tunnel: "LAB01-1" -> [w712 w714]
                          frame #0 {
                            n517 = call "sub vi - defrag tdms v1.vi"("panel id"=w712) -> ("error out"=w711:errorcluster)  [unwired: 10 in]
                            n518 = local write "data file error"(w711) -> ()
                          }
                          frame #1 {
                            n519 = call "Save data file (stop) v3.vi"("panel id"=w714) -> ("network file save error"=w713:errorcluster)  [unwired: 9 in, 1 out]
                            n520 = local write "RESULT LAB01-1"(FALSE) -> ()
                            n521 = local write "data file error"(w713) -> ()
                          }
                        }
                      }
                    }
                  }
                  frame True {
                    n522 = stacked-sequence {
                      seq-local: [w728 _] -> [_ w732]
                      tunnel: w726 -> [_ w742]
                      tunnel: w725 -> [_ w741]
                      tunnel: w724 -> [_ w740]
                      tunnel: w723 -> [_ w739]
                      tunnel: w722 -> [_ w738]
                      tunnel: [_ w737] -> w721
                      tunnel: w720 -> [_ w736]
                      tunnel: w719 -> [_ w735]
                      tunnel: w718 -> [_ w734]
                      tunnel: w717 -> [w730 w733]
                      tunnel: w716 -> [_ w731]
                      frame #0 {
                        n523 = Unbundle(w730) -> ("AMPS"=w729:dbl)  [unwired: 4 out]
                        n524 = call "Check For Amps on v1.vi"("ID"="LAB01-1", "amps"=w729) -> ("amps"=w728:bool)  [unwired: 9 in]
                      }
                      frame #1 {
                        n525 = case shown="True" w732 {
                          tunnel: w742 -> [_ w755]
                          tunnel: w741 -> [_ w754]
                          tunnel: w740 -> [_ w753]
                          tunnel: w739 -> [_ w752]
                          tunnel: w738 -> [_ w751]
                          tunnel: [errorcluster {"status"=FALSE, "code"=0, "source"=""} ("error out") w750] -> w737
                          tunnel: w736 -> [_ w749]
                          tunnel: w735 -> [_ w748]
                          tunnel: w734 -> [_ w747]
                          tunnel: w733 -> [_ w746]
                          tunnel: w731 -> [_ w745]
                          frame False {
                            w743 = FALSE
                            n526 = local write "RUN LAB01-1"(w743) -> ()
                            n527 = local write "run lab01-1"(w743) -> ()
                          }
                          frame True {
                            n528 = stacked-sequence {
                              seq-local: [w756 _ _ _ _] -> [_ w777 _ _ _]
                              tunnel: w755 -> [w761 _ _ _ _]
                              tunnel: w754 -> [w757 _ _ _ _]
                              tunnel: w753 -> [w771 _ _ _ _]
                              tunnel: w752 -> [w764 _ _ _ _]
                              tunnel: w751 -> [w759 _ _ _ _]
                              tunnel: [_ w778 _ _ _] -> w750
                              tunnel: w749 -> [_ _ _ w799 _]
                              tunnel: w748 -> [_ _ _ w809 _]
                              tunnel: w747 -> [_ _ _ w808 _]
                              tunnel: w746 -> [_ _ _ _ _]
                              tunnel: w745 -> [_ _ _ _ w815]
                              frame #0 {
                                w758 = "\\"
                                n529 = case shown="\"CHART TEST\", Default" w771 {
                                tunnel: ["L01-1-CHART TEST-" "L01-1-CYCLE TEST-" "L01-1-T-RISE TEST-"] -> w767
                                frame "CHART TEST", Default {
                                }
                                frame "CYCLE TEST" {
                                }
                                frame "T-RISE TEST" {
                                }
                                }
                                n530 = local read "SET LAB01-1"() -> (w766:T5)
                                n531 = Unbundle(w766) -> ("DESCRIPTION"=w765:string)  [unwired: 4 out]
                                n532 = Concatenate Strings(w761, "\\", w759, w758, w757, w758) -> (w768:string)
                                n533 = String To Path(string=w768) -> (path=w770:path)
                                n534 = Concatenate Strings(w768, w767, w765, "-", w764, ".tdms") -> (w756:string)
                                n535 = Create Folder(path (use dialog)=w770) -> (error out=w769:errorcluster)  [unwired: 2 in, 2 out]
                                n536 = call <vilib>:"Clear Errors.vi"("error in (no error)"=w769) -> ()  [unwired: 5 in, 2 out]
                                n537 = global write "Global 1.vi" "LAB01-1 FILE"(w756) -> ()
                              }
                              frame #1 {
                                (unwired) FALSE
                                n538 = String To Path(string=w777) -> (path=w775:path)
                                n539 = TDMS Open(6:FALSE, 10:T21."create or replace" ("operation (0:open)"), 11:w775) -> (0:w778:errorcluster, 3:→"TDMS LAB01-1":refnum<k34>)  [unwired: 4 in]
                              }
                              frame #2 {
                                n540 = local read "TDMS LAB01-1"() -> (w797:refnum<k34>)
                                n541 = local read "SET LAB01-1"() -> (w786:T5)
                                n542 = Build Array("Testers Name", "Description", "Set Test Cycles", "T-Rise minutes", "T-Rise Deg C") -> (w787:string[])
                                n543 = Unbundle(w786) -> ("NAME"=w785:string, "DESCRIPTION"=w784:string, "CYCLES"=w783:dbl, "T-RISE mins"=w782:dbl, "T-RISE deg C"=w781:dbl)
                                n544 = Number To Decimal String(number=w783) -> (decimal integer string=w796:string)  [unwired: 1 in]
                                n545 = Number To Decimal String(number=w782) -> (decimal integer string=w795:string)  [unwired: 1 in]
                                n546 = Number To Decimal String(number=w781) -> (decimal integer string=w794:string)  [unwired: 1 in]
                                n547 = Build Array(w785, w784, w796, w795, w794) -> (w793:string[])
                                n548 = TDMS Set Properties(5:w793, 7:w787, 11:w797) -> ()  [unwired: 3 in, 4 out]
                              }
                              frame #3 {
                                n549 = local read "DISP LAB01-1"() -> (w807:T4)
                                n550 = Concatenate Strings("LAB01-1  ", w799) -> (w798:string)
                                n551 = Two Button Dialog(message=w798, 1:w808, 2:w809) -> (T button?=w801:bool)
                                n552 = case shown="True" w801 {
                                tunnel: w807 -> [w812 w813]
                                tunnel: [w812 w813] -> w806
                                tunnel: [w811 w814] -> w805
                                tunnel: [w810 w814] -> w804
                                frame False {
                                n553 = Unbundle(w812) -> ("CYCLE"=w811:dbl, "MINS"=w810:dbl)  [unwired: 1 out]
                                }
                                frame True {
                                w814 = 0.0
                                }
                                }
                                n554 = Bundle(cluster=w806, "CYCLE"=w805, "MINS"=w804, "STATUS"="RUN") -> (w803:T4)
                                n555 = local write "DISP LAB01-1"(w803) -> ()
                              }
                              frame #4 {
                                n556 = local read "TEMP START LAB01-1"() -> (w817:cluster{"TL":dbl, "TN":dbl})
                                n557 = Bundle(cluster=w817, "TL"=w815, "TN"=w815) -> (w816:cluster{"TL":dbl, "TN":dbl})
                                n558 = local write "TEMP START LAB01-1"(w816) -> ()
                              }
                            }
                          }
                        }
                      }
                    }
                  }
                }
              }
              event "RUN LAB01-2": Value Change {
                n559 = event-data() -> ("NewVal"=w822:bool)  [unwired: 1 in, 5 out]
                n560 = local write "run lab01-2"(w822) -> ()
                n561 = case shown="True" w822 {
                  tunnel: w828 -> [_ w866]
                  tunnel: w827 -> [_ w865]
                  tunnel: w825 -> [w830 w864]
                  tunnel: w826 -> [_ w863]
                  tunnel: w824 -> [_ w862]
                  tunnel: [w829 w861] -> w823
                  tunnel: w821 -> [_ w860]
                  tunnel: w820 -> [_ w859]
                  tunnel: w819 -> [_ w858]
                  tunnel: w818 -> [_ w856]
                  frame False {
                    # "stop test"
                    n562 = stacked-sequence {
                      tunnel: w830 -> [w839 _]
                      tunnel: [w831 _] -> w829
                      frame #0 {
                        n563 = local read "DISP LAB01-2"() -> (w838:T4)
                        n564 = Unbundle(w838) -> ("CYCLE"=w836:dbl, "MINS"=w837:dbl)  [unwired: 1 out]
                        n565 = case shown="\"CHART TEST\", Default" w839 {
                          tunnel: w837 -> [_ _ w846]
                          tunnel: w836 -> [w844 w845 _]
                          tunnel: [w844 w845 w846] -> w835
                          frame "CHART TEST", Default {
                          }
                          frame "CYCLE TEST" {
                          }
                          frame "T-RISE TEST" {
                          }
                        }
                        n566 = local read "TDMS LAB01-2"() -> (w843:refnum<k34>)
                        n567 = Build Array("STOPPED") -> (w840:string[])
                        n568 = Build Array(w835) -> (w834:dbl[])
                        n569 = TDMS Write(0:w843, 5:"TEST RESULT", 7:w840, 9:w834) -> (4:w832:refnum<k34>, 15:w833:errorcluster)  [unwired: 2 in, 2 out]
                        n570 = TDMS Close(8:w833, 11:w832) -> (0:w831:errorcluster)  [unwired: 1 out]
                      }
                      frame #1 {
                        n571 = local read "DISP LAB01-2"() -> (w850:T4)
                        n572 = stacked-sequence {
                          tunnel: "LAB01-2" -> [w852 w854]
                          frame #0 {
                            n573 = call "sub vi - defrag tdms v1.vi"("panel id"=w852) -> ("error out"=w851:errorcluster)  [unwired: 10 in]
                            n574 = local write "data file error"(w851) -> ()
                          }
                          frame #1 {
                            n575 = call "Save data file (stop) v3.vi"("panel id"=w854) -> ("network file save error"=w853:errorcluster)  [unwired: 9 in, 1 out]
                            n576 = local write "RESULT LAB01-2"(FALSE) -> ()
                            n577 = local write "data file error"(w853) -> ()
                          }
                        }
                        n578 = Bundle(cluster=w850, "STATUS"="STOP") -> (w848:T4)  [unwired: 2 in]
                        n579 = local write "DISP LAB01-2"(w848) -> ()
                      }
                    }
                  }
                  frame True {
                    n580 = local read "SIG LAB01-2"() -> (w857:T2)
                    n581 = stacked-sequence {
                      seq-local: [w868 _] -> [_ w872]
                      tunnel: w866 -> [_ w882]
                      tunnel: w865 -> [_ w881]
                      tunnel: w864 -> [_ w880]
                      tunnel: w863 -> [_ w879]
                      tunnel: w862 -> [_ w878]
                      tunnel: [_ w877] -> w861
                      tunnel: w860 -> [_ w876]
                      tunnel: w859 -> [_ w875]
                      tunnel: w858 -> [_ w874]
                      tunnel: w857 -> [w867 w873]
                      tunnel: w856 -> [_ w871]
                      frame #0 {
